vi "zeroes.vi"   [LabVIEW 2020, in "NI_Gmath.lvlib"]
uses:
  NI_Gmath.lvlib
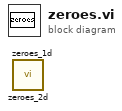
[diagram p0: block diagram]
diagram:
  n1 = call "zeroes_2d.vi"() -> ()  [unwired: 8 in, 1 out]
  n2 = call "zeroes_1d.vi"() -> ()  [unwired: 8 in, 1 out]
